vi "ReadMotorEncoderUsingSdoRead.vi"(8 "error in (no error)":errorcluster, 11 "CANopen Session In":refnum<class "sbCANopenBaseClass.lvclass">) -> (2 "ReadValues":i32[](array[numeric]))   [LabVIEW 2024]
uses:
  <vilib>/addons/Maxon Motor/EPOS2 CANopen/CANopen/sbCANopenBaseClass.lvclass
  <vilib>/addons/Maxon Motor/EPOS2 CANopen/EPOS2 Support Files/Typedefs/EPOS2 PDO Object Data.ctl
  <vilib>/addons/Maxon Motor/EPOS2 CANopen/EPOS2 Library.lvlib
panel:
  out "error out 3":errorcluster
  out "Data 3":u8[](array[numeric])
  out "Position(qc)":i32
  out "error out 2":errorcluster
  out "Data 2":u8[](array[numeric])
  out "Veloxity(rpm)":i32
  out "Current(mA)":i32
  out "Data":u8[](array[numeric])
  out "error out":errorcluster
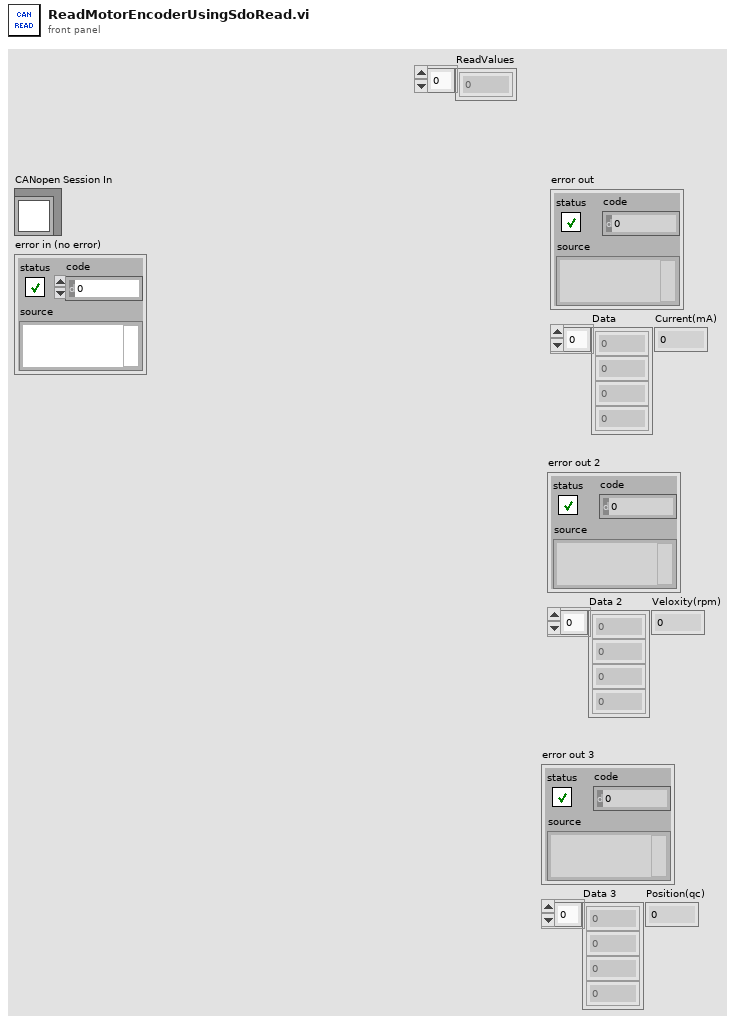
[diagram p1: front panel]
types:
  T1 = typedef "EPOS2 Library.lvlib/EPOS2 PDO Object Data.ctl" = cluster{"Index":u16, "Sub Index":u8, "Size":u8}
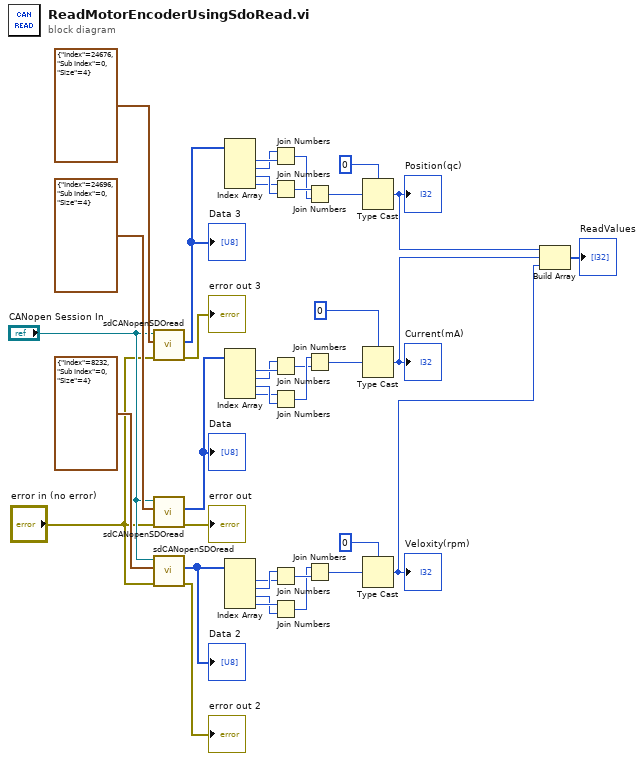
[diagram p0: block diagram]
diagram:
  n1 = call-dynamic "sdCANopenSDOread.vi"("error in (no error)"="error in (no error)", "SDO Read Data"=T1 {"Index"=24676, "Sub Index"=0, "Size"=4} ("PDO Object Data"), "sbCANopenBaseClass in"="CANopen Session In") -> ("error out"=→"error out 3":errorcluster, "Data"=w14:u8[])  [unwired: 6 in, 1 out]
  "Data 3" <- w14
  n2 = call-dynamic "sdCANopenSDOread.vi"("error in (no error)"="error in (no error)", "SDO Read Data"=T1 {"Index"=24696, "Sub Index"=0, "Size"=4} ("PDO Object Data"), "sbCANopenBaseClass in"="CANopen Session In") -> ("error out"=→"error out":errorcluster, "Data"=w36:u8[])  [unwired: 6 in, 1 out]
  "Data" <- w36
  n3 = call-dynamic "sdCANopenSDOread.vi"("error in (no error)"="error in (no error)", "SDO Read Data"=T1 {"Index"=8232, "Sub Index"=0, "Size"=4} ("PDO Object Data"), "sbCANopenBaseClass in"="CANopen Session In") -> ("error out"=→"error out 2":errorcluster, "Data"=w23:u8[])  [unwired: 6 in, 1 out]
  "Data 2" <- w23
  n4 = Index Array(array=w14) -> (element #1=w13:u8, element #2=w12:u8, element #3=w11:u8, element #4=w10:u8)  [unwired: 4 in]
  n5 = Index Array(array=w36) -> (element #1=w35:u8, element #2=w34:u8, element #3=w33:u8, element #4=w32:u8)  [unwired: 4 in]
  n6 = Index Array(array=w23) -> (element #1=w24:u8, element #2=w25:u8, element #3=w26:u8, element #4=w27:u8)  [unwired: 4 in]
  n7 = Join Numbers(hi=w12, lo=w13) -> ((hi.lo)=w8:u16)
  n8 = Join Numbers(hi=w10, lo=w11) -> ((hi.lo)=w9:u16)
  n9 = Join Numbers(hi=w34, lo=w35) -> ((hi.lo)=w30:u16)
  n10 = Join Numbers(hi=w32, lo=w33) -> ((hi.lo)=w31:u16)
  n11 = Join Numbers(hi=w25, lo=w24) -> ((hi.lo)=w29:u16)
  n12 = Join Numbers(hi=w27, lo=w26) -> ((hi.lo)=w28:u16)
  n13 = Join Numbers(hi=w9, lo=w8) -> ((hi.lo)=w15:u32)
  n14 = Join Numbers(hi=w31, lo=w30) -> ((hi.lo)=w37:u32)
  n15 = Join Numbers(hi=w28, lo=w29) -> ((hi.lo)=w22:u32)
  n16 = Type Cast(type=0, x=w15) -> (*(type *) &x=w5:i32)
  "Position(qc)" <- w5
  n17 = Type Cast(type=0, x=w37) -> (*(type *) &x=w4:i32)
  "Current(mA)" <- w4
  n18 = Type Cast(type=0, x=w22) -> (*(type *) &x=w3:i32)
  "Veloxity(rpm)" <- w3
  n19 = Build Array(w5, w4, w3) -> (→"ReadValues":i32[])
